vi "RGB-HSV.vi"(7 "RGB":cluster{"R":sgl, "G":sgl, "B":sgl}) -> (10 "HSV":cluster{"H":sgl, "S":sgl, "V":sgl}, 15 "YUV":cluster{"Y":sgl, "U":sgl, "V":sgl})   [LabVIEW 2014]
doc: "Converts the RGB (Red Green Blue) input to HSV (Hue/Saturation/Value) and YUV (Luminance/Blue/Red) outputs. YUV is used interchangeably with YCbCr.\n\n\nModified for Benilde St. Margaret's School - Tim Jump\nBy Doug Schmertman - Logic PD\nCopyright 2012"
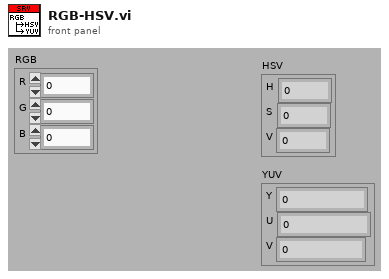
[diagram p1: front panel]
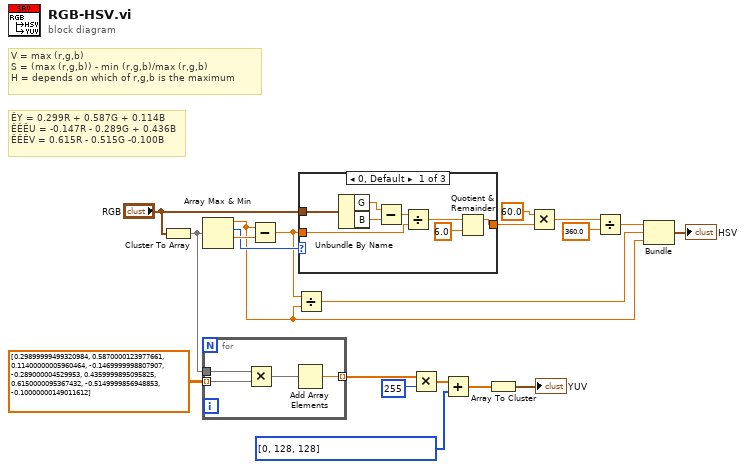
[diagram p0: block diagram]
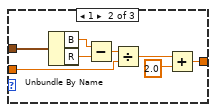
[diagram p2: hidden frame]
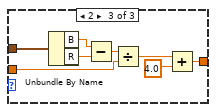
[diagram p3: hidden frame]
diagram:
  # "ÊY = 0.299R + 0.587G + 0.114B\nÊÊÊU = -0.147R - 0.289G + 0.436B\nÊÊÊV = 0.615R - 0.515G -0.100B"
  # "V = max (r,g,b)\nS = (max (r,g,b)) - min (r,g,b)/max (r,g,b)\nH = depends on which of r,g,b is the maximum"
  n1 = Cluster To Array(cluster="RGB") -> (array=w7:sgl[])
  n2 = Array Max & Min(array=w7) -> (max value=w14:sgl, max index (indices)=w19:i32, min value=w20:sgl)  [unwired: 1 out]
  n3 = for {
    tunnel: sgl[][] [[0.299, 0.587, 0.114], [-0.147, -0.289, 0.436], [0.615, -0.515, -0.1]] -> [w24] mode=indexing
    tunnel: w7 -> [w23]
    tunnel: [w21] -> w5 mode=indexing
    n4 = Multiply(x=w23, y=w24) -> (x*y=w22:sgl[])
    n5 = Add Array Elements(numeric array=w22) -> (sum=w21:sgl)
  }
  n6 = Subtract(x=w14, y=w20) -> (x-y=w15:sgl)
  n7 = Divide(x=w15, y=w14) -> (x/y=w16:sgl)
  n8 = case shown="0, Default" w19 {
    tunnel: "RGB" -> [w32 w40 w48]
    tunnel: w15 -> [w28 w36 w44]
    tunnel: [w25 w33 w41] -> w13
    frame 0, Default {
      n9 = Unbundle By Name(w32) -> ("G"=w31:sgl, "B"=w30:sgl)
      n10 = Subtract(x=w31, y=w30) -> (x-y=w29:sgl)
      n11 = Divide(x=w29, y=w28) -> (x/y=w27:sgl)
      n12 = Quotient & Remainder(x=w27, y=sgl 6.0) -> (x-y*floor(x/y)=w25:sgl)  [unwired: 1 out]
    }
    frame 1 {
      n13 = Unbundle By Name(w40) -> ("B"=w39:sgl, "R"=w38:sgl)
      n14 = Subtract(x=w39, y=w38) -> (x-y=w37:sgl)
      n15 = Divide(x=w37, y=w36) -> (x/y=w35:sgl)
      n16 = Add(x=w35, y=sgl 2.0) -> (x+y=w33:sgl)
    }
    frame 2 {
      n17 = Unbundle By Name(w48) -> ("B"=w47:sgl, "R"=w46:sgl)
      n18 = Subtract(x=w47, y=w46) -> (x-y=w45:sgl)
      n19 = Divide(x=w45, y=w44) -> (x/y=w43:sgl)
      n20 = Add(x=w43, y=sgl 4.0) -> (x+y=w41:sgl)
    }
  }
  n21 = Multiply(x=w5, y=i16 255) -> (x*y=w2:sgl[])
  n22 = Add(x=w2, y=u8[] [0, 128, 128]) -> (x+y=w1:sgl[])
  n23 = Array To Cluster(array=w1) -> (cluster=→"YUV":cluster{"[0]":sgl, "[1]":sgl, "[2]":sgl})
  n24 = Multiply(x=sgl 60.0 ("y"), y=w13) -> (x*y=w11:sgl)
  n25 = Divide(x=w11, y=sgl 360.0) -> (x/y=w9:sgl)
  n26 = Bundle(w9, w16, w14) -> (→"HSV":cluster{sgl, sgl, sgl})  [unwired: 1 in]
